vi "Read Type.vi"(8 "Error In":errorcluster, 11 "Datum In":refnum<class "Path.lvclass">) -> (0 "Error Out":errorcluster, 2 "Type":T1=enum."Path", 3 "Datum Out":refnum<class "Path.lvclass">)   [LabVIEW 2018, in "Toolkit.lvlib" / "Data.lvlib" / "Path.lvclass"]
doc: "Get the Mustache data type of an object."
uses:
  Path.lvclass
  Type Defintions/Types.ctl
  Data.lvlib
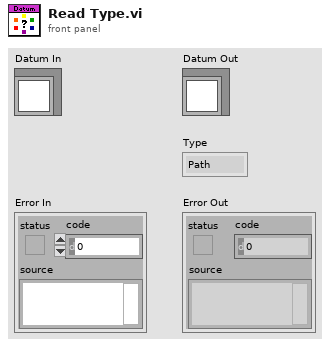
[diagram p1: front panel]
types:
  T1 = typedef "Toolkit.lvlib/Data.lvlib/Types.ctl" = enum16{"Array", "Boolean", "Function", "Map", "Null", "Pair", "Path", "String", "Unknown"}
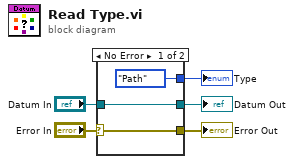
[diagram p0: block diagram]
diagram:
  n1 = case shown="No Error" "Error In" {
    selector: "Error In" -> [w8 w9]
    tunnel: [w8 w9] -> w4
    tunnel: "Datum In" -> [w7 w10]
    tunnel: [w7 w10] -> w2
    tunnel: [Types."Path" ("Type") _] -> w1
    frame No Error {
    }
    frame Error {
    }
  }
  "Error Out" <- w4
  "Datum Out" <- w2
  "Type" <- w1
